vi "Sequence Editor.vi"() -> ()   [LabVIEW 2013, in "Simple Sequence Editor.lvlib"]
uses:
  Simple Sequence Editor.lvlib
  Types/UI.PropertiesTypes.ctl
  Types/StateVariables.ctl
  Types/ChannelProperties.ctl
panel:
  in  "Sequence":i32[](listbox)
  in  "Iteration Information Channel":string(combo)
  in  "Iterations":u32=1 min=1
  in  "View":T1=enum."Sequence Properties"
  in  "Abort Channel":string(combo)
  in  "Step Information Channel":string(combo)
  out "Graph":waveform(dbl)[](graph)
  out "Path":path
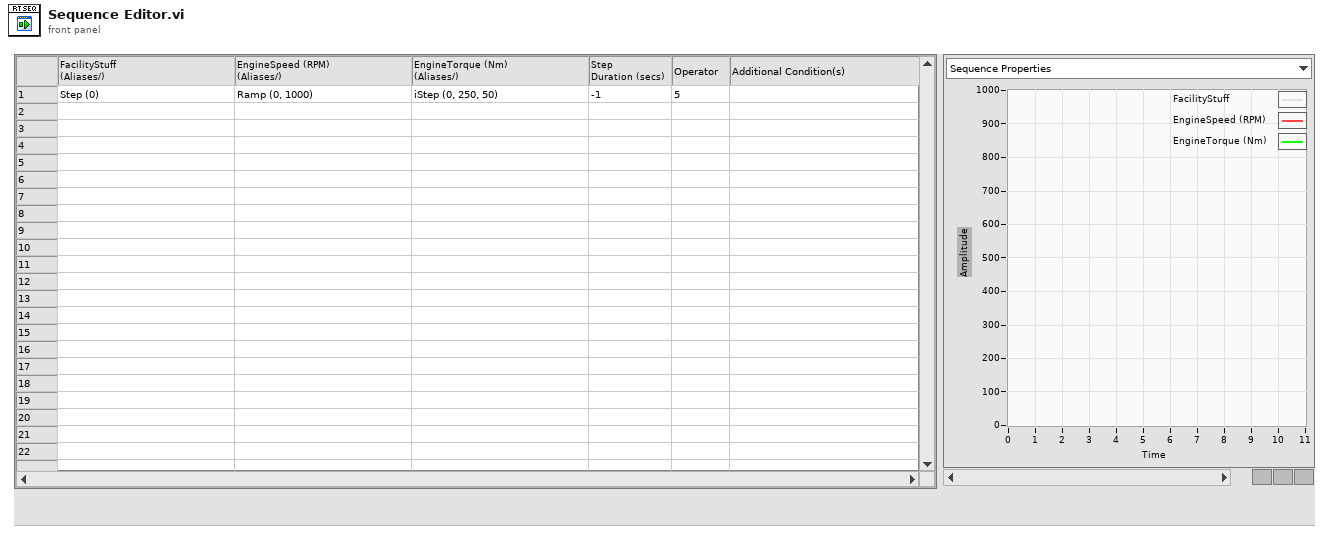
[diagram p1: front panel]
types:
  T1 = typedef "Simple Sequence Editor.lvlib/UI.PropertiesTypes.ctl" = enum8{"Step Properties", "Sequence Properties"}
  T2 = typedef "Simple Sequence Editor.lvlib/StateVariables.ctl" = cluster{"Aliases.All":T3[], "Aliases.Outputs":T3[], "UI.Sequence#ofColumns":i32, "SysDef.Path":path, "UI.SequenceRef":refnum<vi>, "UI.StepInformationRef":refnum<vi>, "UI.AbortRef":refnum<vi>, "UI.GraphRef":refnum<vi>, "UI.ViewRef":refnum<vi>, "UI.IterationsRef":refnum<vi>, "UI.IterationInformationRef":refnum<vi>}
  T3 = typedef "Simple Sequence Editor.lvlib/ChannelProperties.ctl" = cluster{"Name":string, "NodePath":string, "ScaleUnits":string}
  T4 = typedef "LVPoint32TypeDef.ctl" = cluster{"Horizontal":i32, "Vertical":i32}
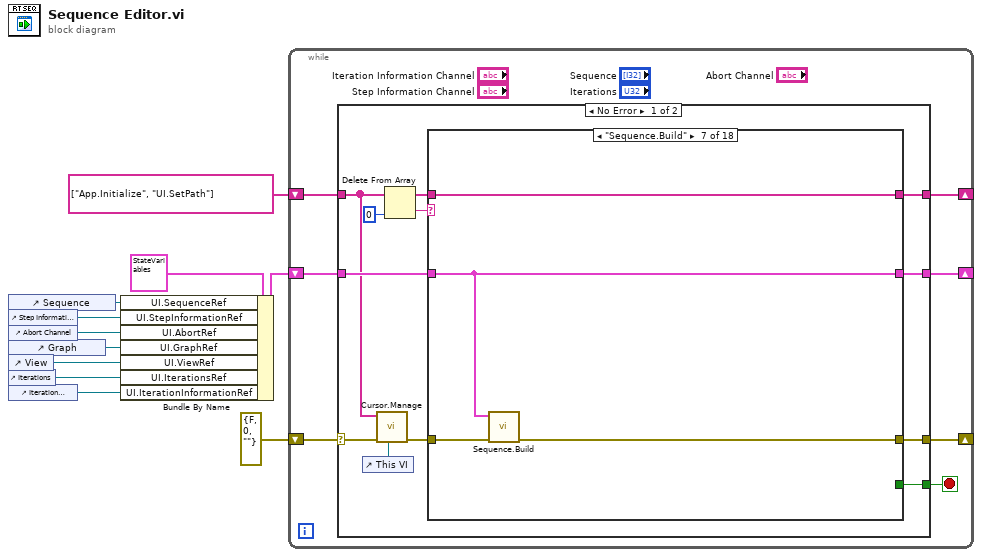
[diagram p0: block diagram]
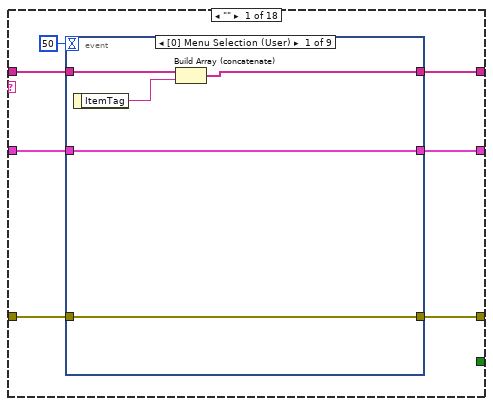
[diagram p2: hidden frame]
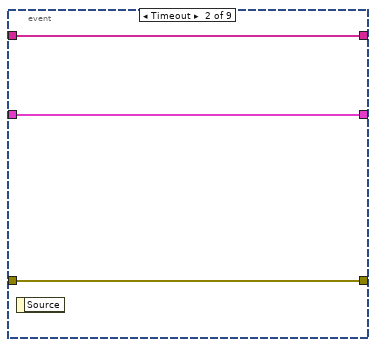
[diagram p3: hidden frame]
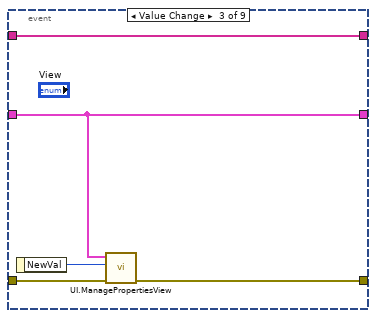
[diagram p4: hidden frame]
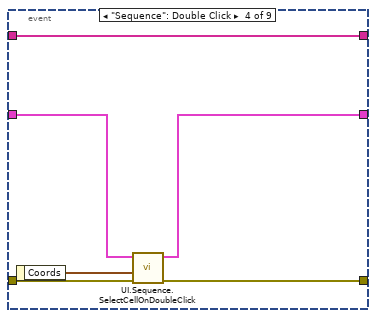
[diagram p5: hidden frame]
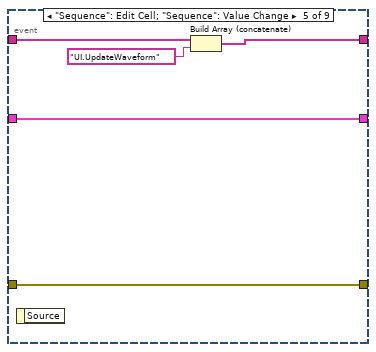
[diagram p6: hidden frame]
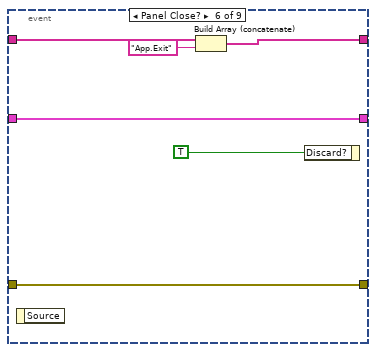
[diagram p7: hidden frame]
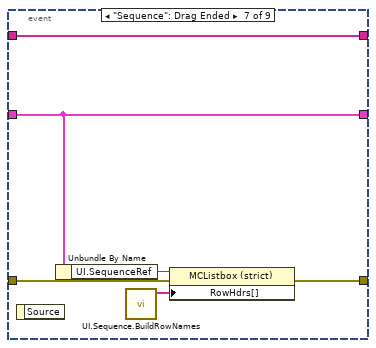
[diagram p8: hidden frame]
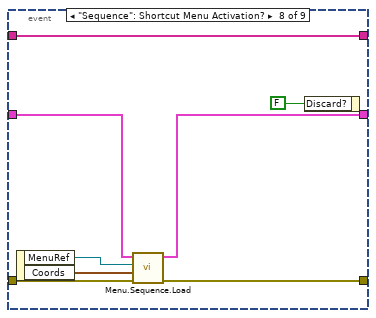
[diagram p9: hidden frame]
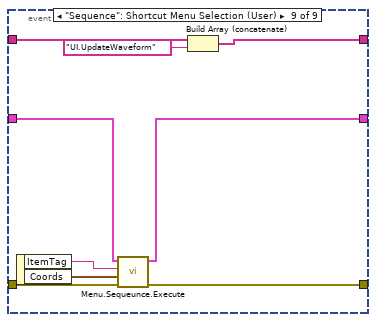
[diagram p10: hidden frame]
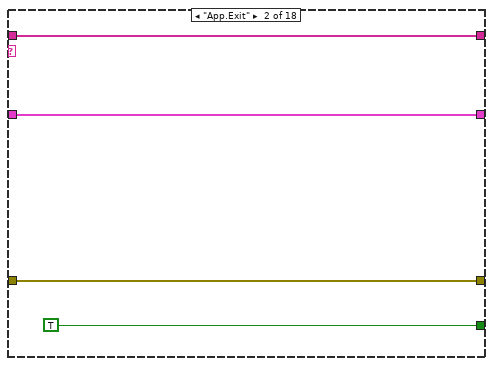
[diagram p11: hidden frame]
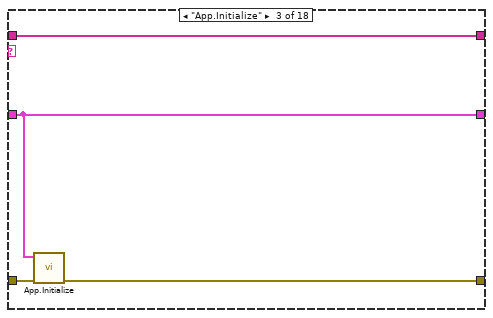
[diagram p12: hidden frame]
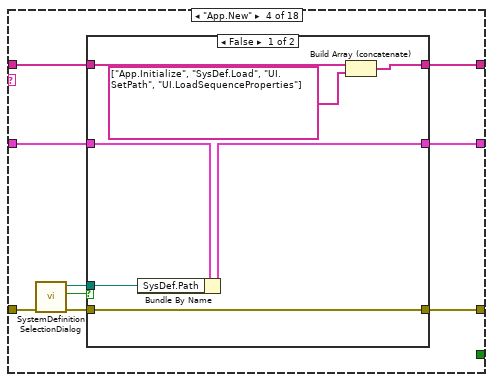
[diagram p13: hidden frame]
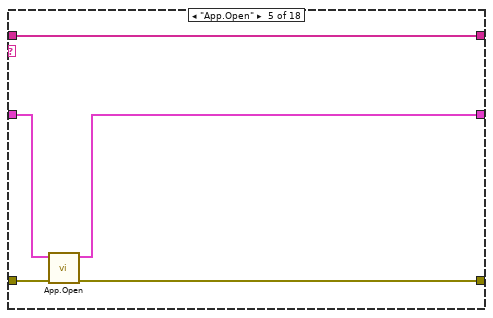
[diagram p15: hidden frame]
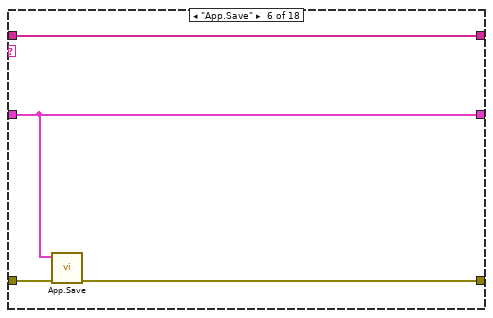
[diagram p16: hidden frame]
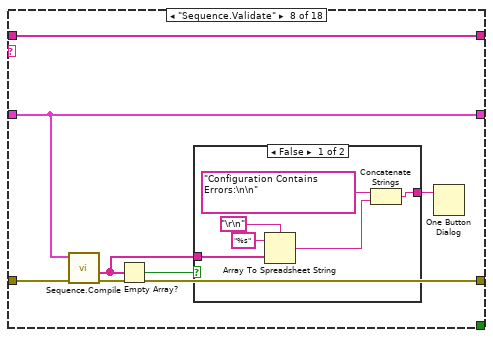
[diagram p17: hidden frame]
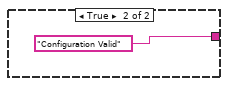
[diagram p18: hidden frame]
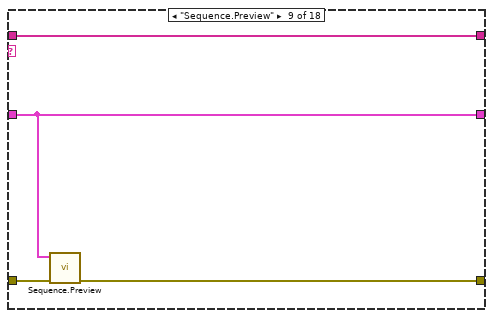
[diagram p19: hidden frame]
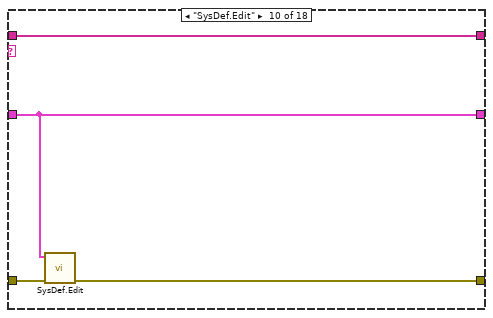
[diagram p20: hidden frame]
diagram:
  n1 = control-ref of="Sequence"() -> (w7:refnum<vi>)
  n2 = control-ref of="Step Information Channel"() -> (w6:refnum<vi>)
  n3 = control-ref of="Abort Channel"() -> (w5:refnum<vi>)
  n4 = control-ref of="Graph"() -> (w4:refnum<vi>)
  n5 = control-ref of="View"() -> (w3:refnum<vi>)
  n6 = control-ref of="Iterations"() -> (w2:refnum<vi>)
  n7 = control-ref of="Iteration Information Channel"() -> (w1:refnum<vi>)
  n8 = Bundle By Name(cluster=T2 {"Aliases.All"=[], "Aliases.Outputs"=[], "UI.Sequence#ofColumns"=0, "SysDef.Path"=path "", "UI.SequenceRef"=refnum, "UI.StepInformationRef"=refnum, "UI.AbortRef"=refnum, "UI.GraphRef"=refnum, "UI.ViewRef"=refnum, "UI.IterationsRef"=refnum, "UI.IterationInformationRef"=refnum}, "UI.SequenceRef"=w7, "UI.StepInformationRef"=w6, "UI.AbortRef"=w5, "UI.GraphRef"=w4, "UI.ViewRef"=w3, "UI.IterationsRef"=w2, "UI.IterationInformationRef"=w1) -> (w8:T2)
  n9 = while {
    shift-right: [w17] -> _
    shift-left: string[] ["App.Initialize", "UI.SetPath"] -> [w18]
    shift-right: [w15] -> _
    shift-left: w8 -> [w16]
    shift-right: [w13] -> _
    shift-left: errorcluster {"status"=FALSE, "code"=0, "source"=""} ("error constant") -> [w14]
    stop <- w12 stop-if-true
    n10 = case shown="No Error" w14 {
      selector: w14 -> [w22 w207]
      tunnel: w18 -> [w23 w210]
      tunnel: [w29 w210] -> w17
      tunnel: w16 -> [w27 w209]
      tunnel: [w26 w209] -> w15
      tunnel: [w25 w206] -> w13
      tunnel: [w24 _] -> w12
      frame No Error {
        n11 = control-ref of="This VI"() -> (w19:refnum<vi>)
        n12 = call "Cursor.Manage.vi"("VI reference (current VI)"=w19, "error in (no error)"=w22, "Cmd list"=w23) -> ("error out"=w21:errorcluster)  [unwired: 8 in]
        n13 = Delete From Array(array=w23, index=0) -> (deleted portion=w30:string, array with subset deleted=w28:string[])  [unwired: 1 in]
        n14 = case shown="\"Sequence.Build\"" w30 {
          tunnel: [w34 w94 w98 w99 w122 w126 w130 w137 w148 w152 w160 w161 w183 w188 w192 w198 w202 w205] -> w29
          tunnel: w28 -> [w33 w94 w98 w100 w122 w126 w130 w137 w148 w152 w160 w162 w184 w188 w192 w198 w202 w205]
          tunnel: w27 -> [w36 w93 w97 w103 w119 w124 w127 w134 w147 w151 w157 w165 w180 w185 w190 w194 w201 w204]
          tunnel: [w37 w93 w97 w101 w118 w124 w127 w134 w147 w151 w156 w163 w180 w185 w190 w195 w201 w204] -> w26
          tunnel: [w31 w92 w95 w104 w120 w125 w129 w135 w145 w149 w158 w166 w181 w186 w191 w196 w199 w203] -> w25
          tunnel: w21 -> [w32 w92 w96 w106 w121 w123 w128 w136 w146 w150 w153 w168 w181 w187 w191 w193 w200 w203]
          tunnel: [_ TRUE _ _ _ _ _ _ _ _ _ _ _ _ _ _ _ _] -> w24
          frame "" {
            n15 = event shown="[0] Menu Selection (User)" {
              selector: _ -> [_ _ _ _ _ _ _ _ _]
              dyn-events: _ -> [_ _ _ _ _ _ _ _ _]
              timeout: 50 -> [_ _ _ _ _ _ _ _ _]
              tunnel: [w39 w45 w50 w56 w58 w63 w73 w81 w83] -> w34
              tunnel: w33 -> [w41 w45 w50 w56 w61 w67 w73 w81 w90]
              tunnel: [w42 w44 w49 w51 w60 w66 w69 w77 w84] -> w37
              tunnel: w36 -> [w42 w44 w49 w52 w60 w66 w69 w76 w85]
              tunnel: [w40 w43 w46 w53 w59 w65 w70 w78 w86] -> w31
              tunnel: w32 -> [w40 w43 w48 w54 w59 w65 w71 w79 w87]
              event Menu Selection (User) {
                n16 = event-data() -> ("ItemTag"=w38:string)  [unwired: 1 in]
                n17 = Build Array (concatenate)(w41, w38) -> (w39:string[])
              }
              event Timeout {
                n18 = event-data() -> ()  [unwired: 1 in, 1 out]
              }
              event Value Change {
                n19 = event-data() -> ("NewVal"=w47:T1)  [unwired: 1 in]
                n20 = call "UI.ManagePropertiesView.vi"("error in (no error)"=w48, "NewVal"=w47, "State Variables"=w49) -> ("error out"=w46:errorcluster)  [unwired: 8 in]
              }
              event "Sequence": Double Click {
                n21 = event-data() -> ("Coords"=w55:T4)  [unwired: 1 in]
                n22 = call "UI.Sequence.SelectCellOnDoubleClick.vi"("error in (no error)"=w54, "Coords"=w55, "State Variables"=w52) -> ("error out"=w53:errorcluster, "State Variables out"=w51:T2)  [unwired: 7 in]
              }
              event "Sequence": Edit Cell; "Sequence": Value Change {
                n23 = event-data() -> ()  [unwired: 1 in, 1 out]
                n24 = Build Array (concatenate)(w61, "UI.UpdateWaveform" ("message")) -> (w58:string[])
              }
              event Panel Close? {
                n25 = event-data() -> ()  [unwired: 1 in, 1 out]
                n26 = Build Array (concatenate)(w67, "App.Exit") -> (w63:string[])
                n27 = event-data("Discard?"=TRUE) -> ()  [unwired: 1 in, 1 out]
              }
              event "Sequence": Drag Ended {
                n28 = event-data() -> ()  [unwired: 1 in, 1 out]
                n29 = Unbundle By Name(w69) -> ("UI.SequenceRef"=w68:refnum<vi>)
                n30 = call "UI.Sequence.BuildRowNames.vi"() -> ("Row Headings"=w72:string[])  [unwired: 11 in]
                n31 = property class="MCListbox (strict)"(reference=w68, error in=w71, "RowHdrs[]"=w72) -> (error out=w70:errorcluster)  [unwired: 1 out]
              }
              event "Sequence": Shortcut Menu Activation? {
                n32 = event-data() -> ("MenuRef"=w74:refnum<k9>, "Coords"=w75:T4)  [unwired: 1 in]
                n33 = call "Menu.Sequence.Load.vi"("error in (no error)"=w79, "Coords"=w75, "MenuRef"=w74, "State Variables"=w76) -> ("error out"=w78:errorcluster, "State Variables out"=w77:T2)  [unwired: 6 in]
                n34 = event-data("Discard?"=FALSE) -> ()  [unwired: 1 in, 1 out]
              }
              event "Sequence": Shortcut Menu Selection (User) {
                n35 = event-data() -> ("ItemTag"=w89:string, "Coords"=w88:T4)  [unwired: 1 in]
                n36 = call "Menu.Sequeunce.Execute.vi"("error in (no error)"=w87, "Coords"=w88, "ItemPath"=w89, "State Variables"=w85) -> ("error out"=w86:errorcluster, "State Variables out"=w84:T2)  [unwired: 6 in]
                n37 = Build Array (concatenate)(w90, "UI.UpdateWaveform" ("message")) -> (w83:string[])
              }
            }
          }
          frame "App.Exit" {
          }
          frame "App.Initialize" {
            n38 = call "App.Initialize.vi"("error in (no error)"=w96, "Start Variables"=w97) -> ("error out"=w95:errorcluster)  [unwired: 9 in]
          }
          frame "App.New" {
            n39 = call "SystemDefinitionSelectionDialog.vi"("error in (no error)"=w106) -> ("error out"=w107:errorcluster, "cancelled"=w105:bool, "selected path"=w102:path)  [unwired: 8 in]
            n40 = case shown="False" w105 {
              tunnel: w107 -> [w114 w116]
              tunnel: [w114 w116] -> w104
              tunnel: w103 -> [w113 w117]
              tunnel: [w112 w117] -> w101
              tunnel: w102 -> [w111 _]
              tunnel: [w110 w115] -> w99
              tunnel: w100 -> [w108 w115]
              frame False {
                n41 = Bundle By Name(cluster=w113, "SysDef.Path"=w111) -> (w112:T2)
                n42 = Build Array (concatenate)(w108, string[] ["App.Initialize", "SysDef.Load", "UI.SetPath", "UI.LoadSequenceProperties"]) -> (w110:string[])
              }
              frame True {
              }
            }
          }
          frame "App.Open" {
            n43 = call "App.Open.vi"("error in (no error)"=w121, "State Variables"=w119) -> ("error out"=w120:errorcluster, "State Variables out"=w118:T2)  [unwired: 8 in]
          }
          frame "App.Save" {
            n44 = call "App.Save.vi"("error in (no error)"=w123, "State Variables"=w124) -> ("error out"=w125:errorcluster)  [unwired: 9 in]
          }
          frame "Sequence.Build" {
            n45 = call "Sequence.Build.vi"("error in (no error)"=w128, "State Variables"=w127) -> ("error out"=w129:errorcluster)  [unwired: 9 in]
          }
          frame "Sequence.Validate" {
            n46 = call "Sequence.Compile.vi"("error in (no error)"=w136, "State Variables"=w134) -> ("error out"=w135:errorcluster, "Warnings"=w131:string[])  [unwired: 7 in, 1 out]
            n47 = Empty Array?(array=w131) -> (empty?=w133:bool)
            n48 = case shown="False" w133 {
              tunnel: [w141 "Configuration Valid"] -> w132
              tunnel: w131 -> [w142 _]
              frame False {
                n49 = Array To Spreadsheet String(delimiter (Tab)="\r\n", array=w142, 3:"%s" ("format string")) -> (spreadsheet string=w140:string)
                n50 = Concatenate Strings("Configuration Contains Errors:\n\n", w140) -> (w141:string)
              }
              frame True {
              }
            }
            n51 = One Button Dialog(message=w132) -> ()  [unwired: 1 in, 1 out]
          }
          frame "Sequence.Preview" {
            n52 = call "Sequence.Preview.vi"("error in (no error)"=w146, "State Variables"=w147) -> ("error out"=w145:errorcluster)  [unwired: 9 in]
          }
          frame "SysDef.Edit" {
            n53 = call "SysDef.Edit.vi"("error in (no error)"=w150, "State Variables"=w151) -> ("error out"=w149:errorcluster)  [unwired: 9 in]
          }
          frame "SysDef.Load" {
            n54 = Unbundle By Name(w157) -> ("SysDef.Path"=w159:path)
            n55 = call "LoadSystemDefinition.vi"("error in (no error)"=w153, "SysDef.Path"=w159) -> ("error out"=w158:errorcluster, "Aliases.Outputs"=w154:T3[], "Aliases.All"=w155:T3[])  [unwired: 7 in]
            n56 = Bundle By Name(cluster=w157, "Aliases.All"=w155, "Aliases.Outputs"=w154) -> (w156:T2)
          }
          frame "SysDef.New" {
            n57 = call "SystemDefinitionSelectionDialog.vi"("error in (no error)"=w168) -> ("error out"=w169:errorcluster, "cancelled"=w167:bool, "selected path"=w164:path)  [unwired: 8 in]
            n58 = case shown="True" w167 {
              tunnel: w169 -> [w176 w178]
              tunnel: [w176 w178] -> w166
              tunnel: w165 -> [w175 w179]
              tunnel: [w174 w179] -> w163
              tunnel: w164 -> [w173 _]
              tunnel: [w172 w177] -> w161
              tunnel: w162 -> [w170 w177]
              frame False {
                n59 = Bundle By Name(cluster=w175, "SysDef.Path"=w173) -> (w174:T2)
                n60 = Build Array (concatenate)(w170, string[] ["SysDef.Load", "UI.SetPath", "UI.LoadSequenceProperties"]) -> (w172:string[])
              }
              frame True {
              }
            }
          }
          frame "SysDef.Refresh" {
            n61 = Build Array (concatenate)(w184, string[] ["SysDef.Load", "UI.SetPath", "UI.LoadSequenceProperties"]) -> (w183:string[])
          }
          frame "Steps.GenerateMultiple" {
            n62 = call "Dialog.MassStepGeneration.vi"("error in (no error)"=w187, "State Variables"=w185) -> ("error out"=w186:errorcluster)  [unwired: 9 in]
          }
          frame "UI.SetPath" {
            n63 = Unbundle By Name(w190) -> ("SysDef.Path"=→"Path":path)
          }
          frame "UI.UpdateWaveform" {
            n64 = call "UI.UpdateWaveform.vi"("error in (no error)"=w193, "State Variables"=w194) -> ("error out"=w196:errorcluster, "Wavefrom"=→"Graph":waveform(dbl)[], "State Variables out"=w195:T2)  [unwired: 7 in]
          }
          frame "UI.LoadSequenceProperties" {
            n65 = call "UI.LoadComboBoxes.vi"("error in (no error)"=w200, "State Variables"=w201) -> ("error out"=w199:errorcluster)  [unwired: 9 in]
          }
          frame Default {
          }
        }
      }
      frame Error {
        n66 = call <vilib>:"Simple Error Handler.vi"("error in (no error)"=w207) -> ("error out"=w208:errorcluster)  [unwired: 4 in, 4 out]
        n67 = call <vilib>:"Clear Errors.vi"("error in (no error)"=w208) -> ("error out"=w206:errorcluster)  [unwired: 6 in]
      }
    }
  }
